vi "SOQPSK Modem.vi"() -> ()   [LabVIEW 2025]
uses:
  chdr/CHDR Header Layout.ctl
  <vilib>/Platform/TimedLoop/XDataNode/timing_clust.ctl
  <vilib>/Platform/TimedLoop/XDataNode/nitl_modes.ctl
  <vilib>/Platform/TimedLoop/XDataNode/wakeup.ctl
  <vilib>/DLsc/v1/FPGA/DLsc/Endpoint/Data Transfer Type.ctl
  <vilib>/DLsc/v1/FPGA/Aurora 64b66b/Aurora Port Identifier.ctl
  Shared/Public/Demodulation Control.ctl
  <vilib>/rvi/Emulation/niFpgaSctlEmulationGetInTimedLoop.vi
  <vilib>/rvi/Emulation/niFpgaEmulationReportErrorSimple.vi
  <vilib>/rvi/Emulation/niFpgaGetClockAttributes.vi
  <vilib>/rvi/Emulation/niFpgaCriticalErrorInLSC.vi
  <vilib>/rvi/Emulation/niFpgaProcessEmulError.vi
  <vilib>/eio/utilities/niEioResolveVilibRelativePath.vi
  <vilib>/rvi/interface/RandomDataEmulation/niFpgaRandomDataHandleErrors.vi
  <vilib>/rvi/Emulation/niFpgaEmulationIsFPGAContextNoSignature.vi
  <vilib>/rvi/errors/niFpgaSetErrorForExecOnDevCompSimple.vi
  <vilib>/rvi/eio/common/nirviEmuReportErrorAndStop.vi
  <vilib>/rvi/DataTransferAndStorage/Container/Common/niFpgaContainerGetUniqueNameForEmu.vi
  <vilib>/rvi/FIFO/Fifo_Resource/nirvififoEmulationSetSize.vi
  <vilib>/rvi/FIFO/Fifo_Resource/nirviFifoEmulationQueueMgr.vi
  <instcachedir>/0/nirviFifoEmulationQueueMgr_E5CAEC123FF24DC58D834DCA3CDAA9B5.lvgen/nirviFifoEmulationQueueMgr_E5CAEC123FF24DC58D834DCA3CDAA9B5_011.vi
  <vilib>/rvi/FIFO/Fifo_Resource/nirvififoEmulationDetermineInputValidOut.vi
  <vilib>/rvi/FIFO/Fifo_Resource/nirvififoEmulationCreateLock.vi
  <vilib>/rvi/FIFO/Fifo_Resource/nirvififoEmulationObtainLock.vi
  <vilib>/rvi/FIFO/Fifo_Resource/nirvififoEmulationReleaseLock.vi
  <vilib>/rvi/occurrence/nirviWaitOnOccurrenceBase.vi
  <vilib>/rvi/errors/nirviReportUnexpectedCaseInternalError.vi
  <vilib>/rvi/errors/nirviReportUnexpectedCaseInternalError (U32).vi
  <vilib>/rvi/interface/RandomDataEmulation/nirviRandomDataMultiElementFPGAFIFO.vi
  <instcachedir>/0/nirviRandomDataMultiElementFPGAFIFO_BE2FF10D3D6E420AB0291A02835C249E.lvgen/nirviRandomDataMultiElementFPGAFIFO_BE2FF10D3D6E420AB0291A02835C249E_001.vi
  <instrlib>/_niInstr/Basic Elements/v1/FPGA/Private/Count Up U32.vi
  <vilib>/rvi/Memory/Memory_Emulation/nirvimemoryFastEmulation.vi
  <vilib>/rvi/Memory/Memory_Emulation/nirvimemoryEmulation.vi
  <vilib>/Utility/error.llb/Clear Errors.vi
  <vilib>/rvi/DataTransferAndStorage/Container/Common/niFpgaContainerSetEmuInfo.vi
  <vilib>/DLsc/v1/FPGA/Aurora 64b66b/Create DX Advanced.vi
  <vilib>/DLsc/v1/FPGA/DLsc/Endpoint/Write Data Stream with Framing 256 Bits.vi
  <vilib>/DLsc/v1/FPGA/DLsc/Endpoint/Read Data Stream with Framing 256 Bits.vi
  <instrlib>/_niInstr/Basic Elements/v1/FPGA/Private/Count Up U64.vi
  <vilib>/Platform/TimedLoop/XDataNode/XDataNode.xnode
  <vilib>/rvi/DataTransferAndStorage/Container/XNode/niFpgaContainer.xnode
  <vilib>/rvi/interface/RandomDataEmulation/nirviRandomDataFpgaReadWriteTemplate.vi
  <vilib>/rvi/FIFO/Fifo_Resource/nirvififoEmulationWrite.vi
  <vilib>/rvi/interface/RandomDataEmulation/nirviRandomDataFpgaMultiElementTemplate.vi
  <vilib>/rvi/FIFO/Fifo_Resource/nirvififoEmulationRead.vi
  <vilib>/rvi/LocalResourceManager/LocalResourceManager.xnode
  <vilib>/DataMovement_sc/v1/FPGA/Buffer U32 8 to 1 SPC/Buffer U32 8 to 1 SPC v1 FPGA.lvclass
  <vilib>/DataMovement_sc/v1/FPGA/Buffer U32 2 to 8 SPC/Buffer U32 2 to 8 SPC v1 FPGA.lvclass
  Shared/BER/FPGA/BER/BER.lvclass
  <vilib>/Platform/TimedLoop/XDataNode/XDNodeRunTimeDep.lvlib
  chdr/CHDR Support.lvlib
  <instrlib>/_niInstr/Basic Elements/v1/FPGA/niInstr Basic Elements v1 FPGA.lvlib
  <vilib>/DataMovement_sc/v1/Shared/Data Types/DMsc Data Types v1 Shared.lvlib
  <instrlib>/_niInstr/FIFO Register Bus/v1/FPGA/niInstr FIFO Register Bus v1 FPGA.lvclass
  <vilib>/DLsc/v1/FPGA/DLsc/Collection/Endpoint Collection.lvclass
  <vilib>/DLsc/v1/FPGA/DLsc/Endpoint/Endpoint.lvclass
  Shared/Modems Shared.lvlib
  Shared/AWGN/FPGA/AWGN FPGA.lvlib
  Shared/SOQPSK Modem Shared.lvlib
  <vilib>/DLsc/v1/FPGA/Aurora 64b66b/DLsc Aurora 64b66b v1 FPGA.lvlib
panel:
  in  "update bit generation.1":bool
  out "last_header.1":T1
  out "last_timestamp.1":u64
  out "error detection.1":T2
  out "header count.1":u64
  in  "reset rx.1":bool
  in  "enable match filter.1":bool
  in  "symmetric filter coefficients .1":T3 {"symmetric filter coefficients[16]" format="%.16g"; "symmetric filter coefficients[0]" format="%.16g"; "symmetric filter coefficients[1]" format="%.16g"; "symmetric filter coefficients[2]" format="%.16g"; "symmetric filter coefficients[3]" format="%.16g"; "symmetric filter coefficients[4]" format="%.16g"; "symmetric filter coefficients[5]" format="%.16g"; "symmetric filter coefficients[6]" format="%.16g"; "symmetric filter coefficients[7]" format="%.16g"; "symmetric filter coefficients[8]" format="%.16g"; "symmetric filter coefficients[9]" format="%.16g"; "symmetric filter coefficients[10]" format="%.16g"; "symmetric filter coefficients[11]" format="%.16g"; "symmetric filter coefficients[12]" format="%.16g"; "symmetric filter coefficients[13]" format="%.16g"; "symmetric filter coefficients[14]" format="%.16g"; "symmetric filter coefficients[15]" format="%.16g"}
  in  "payload length.1":u32
  out "current threshold.1":fxp<+/-,15,15>
  in  "enable aurora debug.1":bool
  in  "preamble.1":i32
  out "demodulated bits overflow.1":bool
  out "aurora debug overflow.1":bool
  out "recovered IQ overflow.1":bool
  in  "demodulation control.1":i16
  out "demodulated bits to BER overflow.1":bool
  out "bit stream length.1":u32
  out "write data stream overflow.1":bool
  in  "reset overflow status.1":bool
  out "modulator error.1":bool
  in  "soqpsk parameters.1":T4
  in  "enable precoder.1":bool
  in  "scaling factor.1":fxp<+,16,0> format="%.16g"
  in  "output type selection.1":u16
  in  "reset modulator.1":bool
  in  "AWGN seeds.1":fxp<+,25,25>[](array[numeric])=[0.0, 0.0]
  in  "enable modulator.1":bool
  in  "header parameters.1":T5
  in  "aurora frame length.1":u16
  in  "reset tx.1":bool
  in  "update bit generation.0":bool
  out "demodulated bits to BER overflow.0":bool
  in  "demodulation control.0":i16
  out "recovered IQ overflow.0":bool
  out "aurora debug overflow.0":bool
  out "demodulated bits overflow.0":bool
  in  "preamble.0":i32
  in  "enable aurora debug.0":bool
  out "current threshold.0":fxp<+/-,15,15>
  in  "payload length.0":u32
  in  "symmetric filter coefficients.0":T3 {"symmetric filter coefficients[16]" format="%.16g"; "symmetric filter coefficients[0]" format="%.16g"; "symmetric filter coefficients[1]" format="%.16g"; "symmetric filter coefficients[2]" format="%.16g"; "symmetric filter coefficients[3]" format="%.16g"; "symmetric filter coefficients[4]" format="%.16g"; "symmetric filter coefficients[5]" format="%.16g"; "symmetric filter coefficients[6]" format="%.16g"; "symmetric filter coefficients[7]" format="%.16g"; "symmetric filter coefficients[8]" format="%.16g"; "symmetric filter coefficients[9]" format="%.16g"; "symmetric filter coefficients[10]" format="%.16g"; "symmetric filter coefficients[11]" format="%.16g"; "symmetric filter coefficients[12]" format="%.16g"; "symmetric filter coefficients[13]" format="%.16g"; "symmetric filter coefficients[14]" format="%.16g"; "symmetric filter coefficients[15]" format="%.16g"}
  in  "enable match filter.0":bool
  in  "enable modulator.0":bool
  in  "AWGN seeds.0":fxp<+,25,25>[](array[numeric])=[0.0, 0.0]
  in  "reset modulator.0":bool
  in  "output type selection.0":u16
  in  "scaling factor.0":fxp<+,16,0> format="%.16g"
  in  "enable precoder.0":bool
  in  "soqpsk parameters.0":T4
  out "modulator error":bool
  in  "reset overflow status.0":bool
  out "write data stream overflow":bool
  out "bit stream length.0":u32
  out "fifo reg bus status 0":u32
  out "fifo reg bus data 0":u64
  in  "fifo reg bus ctrl 0":u32
  in  "reset rx.0":bool
  out "header count.0":u64
  out "error detection.0":T2
  out "last_timestamp.0":u64
  out "last_header.0":T1
  in  "reset tx.0":bool
  in  "aurora frame length.0":u16
  in  "header parameters.0":T5
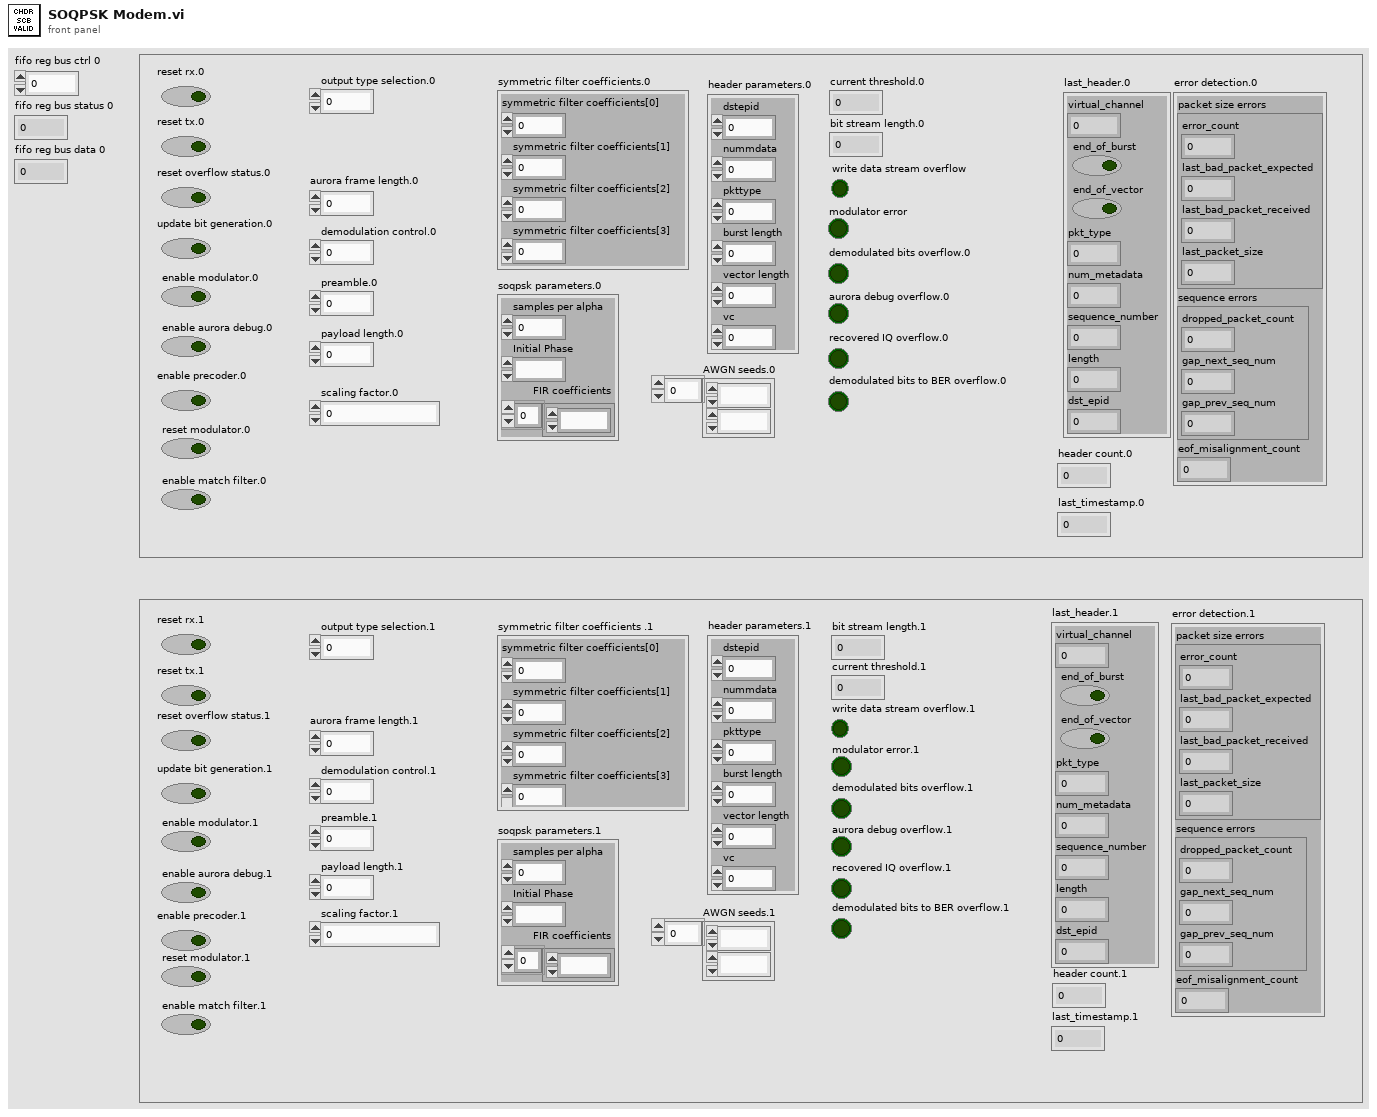
[diagram p1: front panel]
types:
  T1 = typedef "CHDR Support.lvlib/CHDR Header Layout.ctl" = cluster{"virtual_channel":fxp<+,6,6>, "end_of_burst":bool, "end_of_vector":bool, "pkt_type":fxp<+,3,3>, "num_metadata":fxp<+,5,5>, "sequence_number":u16, "length":u16, "dst_epid":u16}
  T2 = cluster{"packet size errors":cluster{"error_count":u64, "last_bad_packet_expected":u16, "last_bad_packet_received":u16, "last_packet_size":u16}, "sequence errors":cluster{"dropped_packet_count":u64, "gap_next_seq_num":u16, "gap_prev_seq_num":u16}, "eof_misalignment_count":u64}
  T3 = cluster{"symmetric filter coefficients[0]":fxp<+/-,16,1>, "symmetric filter coefficients[1]":fxp<+/-,16,1>, "symmetric filter coefficients[2]":fxp<+/-,16,1>, "symmetric filter coefficients[3]":fxp<+/-,16,1>, "symmetric filter coefficients[4]":fxp<+/-,16,1>, "symmetric filter coefficients[5]":fxp<+/-,16,1>, "symmetric filter coefficients[6]":fxp<+/-,16,1>, "symmetric filter coefficients[7]":fxp<+/-,16,1>, "symmetric filter coefficients[8]":fxp<+/-,16,1>, "symmetric filter coefficients[9]":fxp<+/-,16,1>, "symmetric filter coefficients[10]":fxp<+/-,16,1>, "symmetric filter coefficients[11]":fxp<+/-,16,1>, "symmetric filter coefficients[12]":fxp<+/-,16,1>, "symmetric filter coefficients[13]":fxp<+/-,16,1>, "symmetric filter coefficients[14]":fxp<+/-,16,1>, "symmetric filter coefficients[15]":fxp<+/-,16,1>, "symmetric filter coefficients[16]":fxp<+/-,16,1>}
  T4 = cluster{"samples per alpha":u8, "Initial Phase":fxp<+/-,24,1>, "FIR coefficients":fxp<+/-,24,1>[]}
  T5 = cluster{"dstepid":u16, "nummdata":fxp<+,5,5>, "pkttype":fxp<+,3,3>, "burst length":u16, "vector length":u16, "vc":fxp<+,6,6>}
  T6 = typedef "DLsc v1 FPGA.lvlib/Endpoint.lvclass/Data Transfer Type.ctl" = enum16{"u32 1spc", "u32 2spc", "u32 4spc", "u32 8spc", "u32 16spc", "u32 32spc"}
  T7 = typedef "DLsc Aurora 64b66b v1 FPGA.lvlib/Aurora Port Identifier.ctl" = enum16{"Port 0", "Port 1", "Port 2", "Port 3", "Port 4", "Port 5", "Port 6", "Port 7", "Port 8", "Port 9", "Port 10", "Port 11", "Ports 0-1", "Ports 2-3", "Ports 4-5", "Ports 6-7", "Ports 8-9", "Ports 10-11", "Ports 0-3", "Ports 4-7", "Ports 8-11"}
  T8 = typedef "XDNodeRunTimeDep.lvlib/timing_clust.ctl" = cluster{"Expected End [f-1]":u64, "Actual End [f-1]":u64, "Finished Late? [f-1]":bool, "Expected End [i-1]":u64, "Actual End [i-1]":u64, "Finished Late? [i-1]":bool, "Expected Start [i]":u64, "Actual Start [i]":u64, "Expected Start [f]":u64, "Actual Start [f]":u64, "Source Name":string, "Structure Name":string, "Period":i64, "Deadline":i64, "Offset":i64, "Start":i64, "Priority":i32, "Timeout":i32, "Mode":T9, "Wakeup Reason":T10, "Error":errorcluster, "Source Type":string, "Secondary Source Type":string, "Global End Time":u64, "Global Start Time":u64, "Frame Duration":u64, "Iteration Duration":u64, "Assigned CPU":i32, "I/O Scan Engine Mode":u32}
  T9 = typedef "XDNodeRunTimeDep.lvlib/nitl_modes.ctl" = enum32{"No Change", "Process missed periods, maintain original phase", "Discard missed periods, maintain original phase", "Process missed periods, ignore original phase", "Discard missed periods, ignore original phase"}
  T10 = typedef "XDNodeRunTimeDep.lvlib/wakeup.ctl" = enum32{"Normal", "Aborted", "Asynchronous wakeup", "Timing source error", "Timed loop error", "Timeout"}
  T11 = typedef "niInstr DSP v1 Shared.lvlib/IQ Data.ctl" = cluster{"I":fxp<+/-,18,1>, "Q":fxp<+/-,18,1>, "overflow":bool}
  T12 = cluster{"dropped_packet_count":u64, "gap_next_seq_num":u16, "gap_prev_seq_num":u16}
  T13 = cluster{"error_count":u64, "last_bad_packet_expected":u16, "last_bad_packet_received":u16, "last_packet_size":u16}
  T14 = typedef "SOQPSK Modem Shared.lvlib/Demodulation Control.ctl" = i16
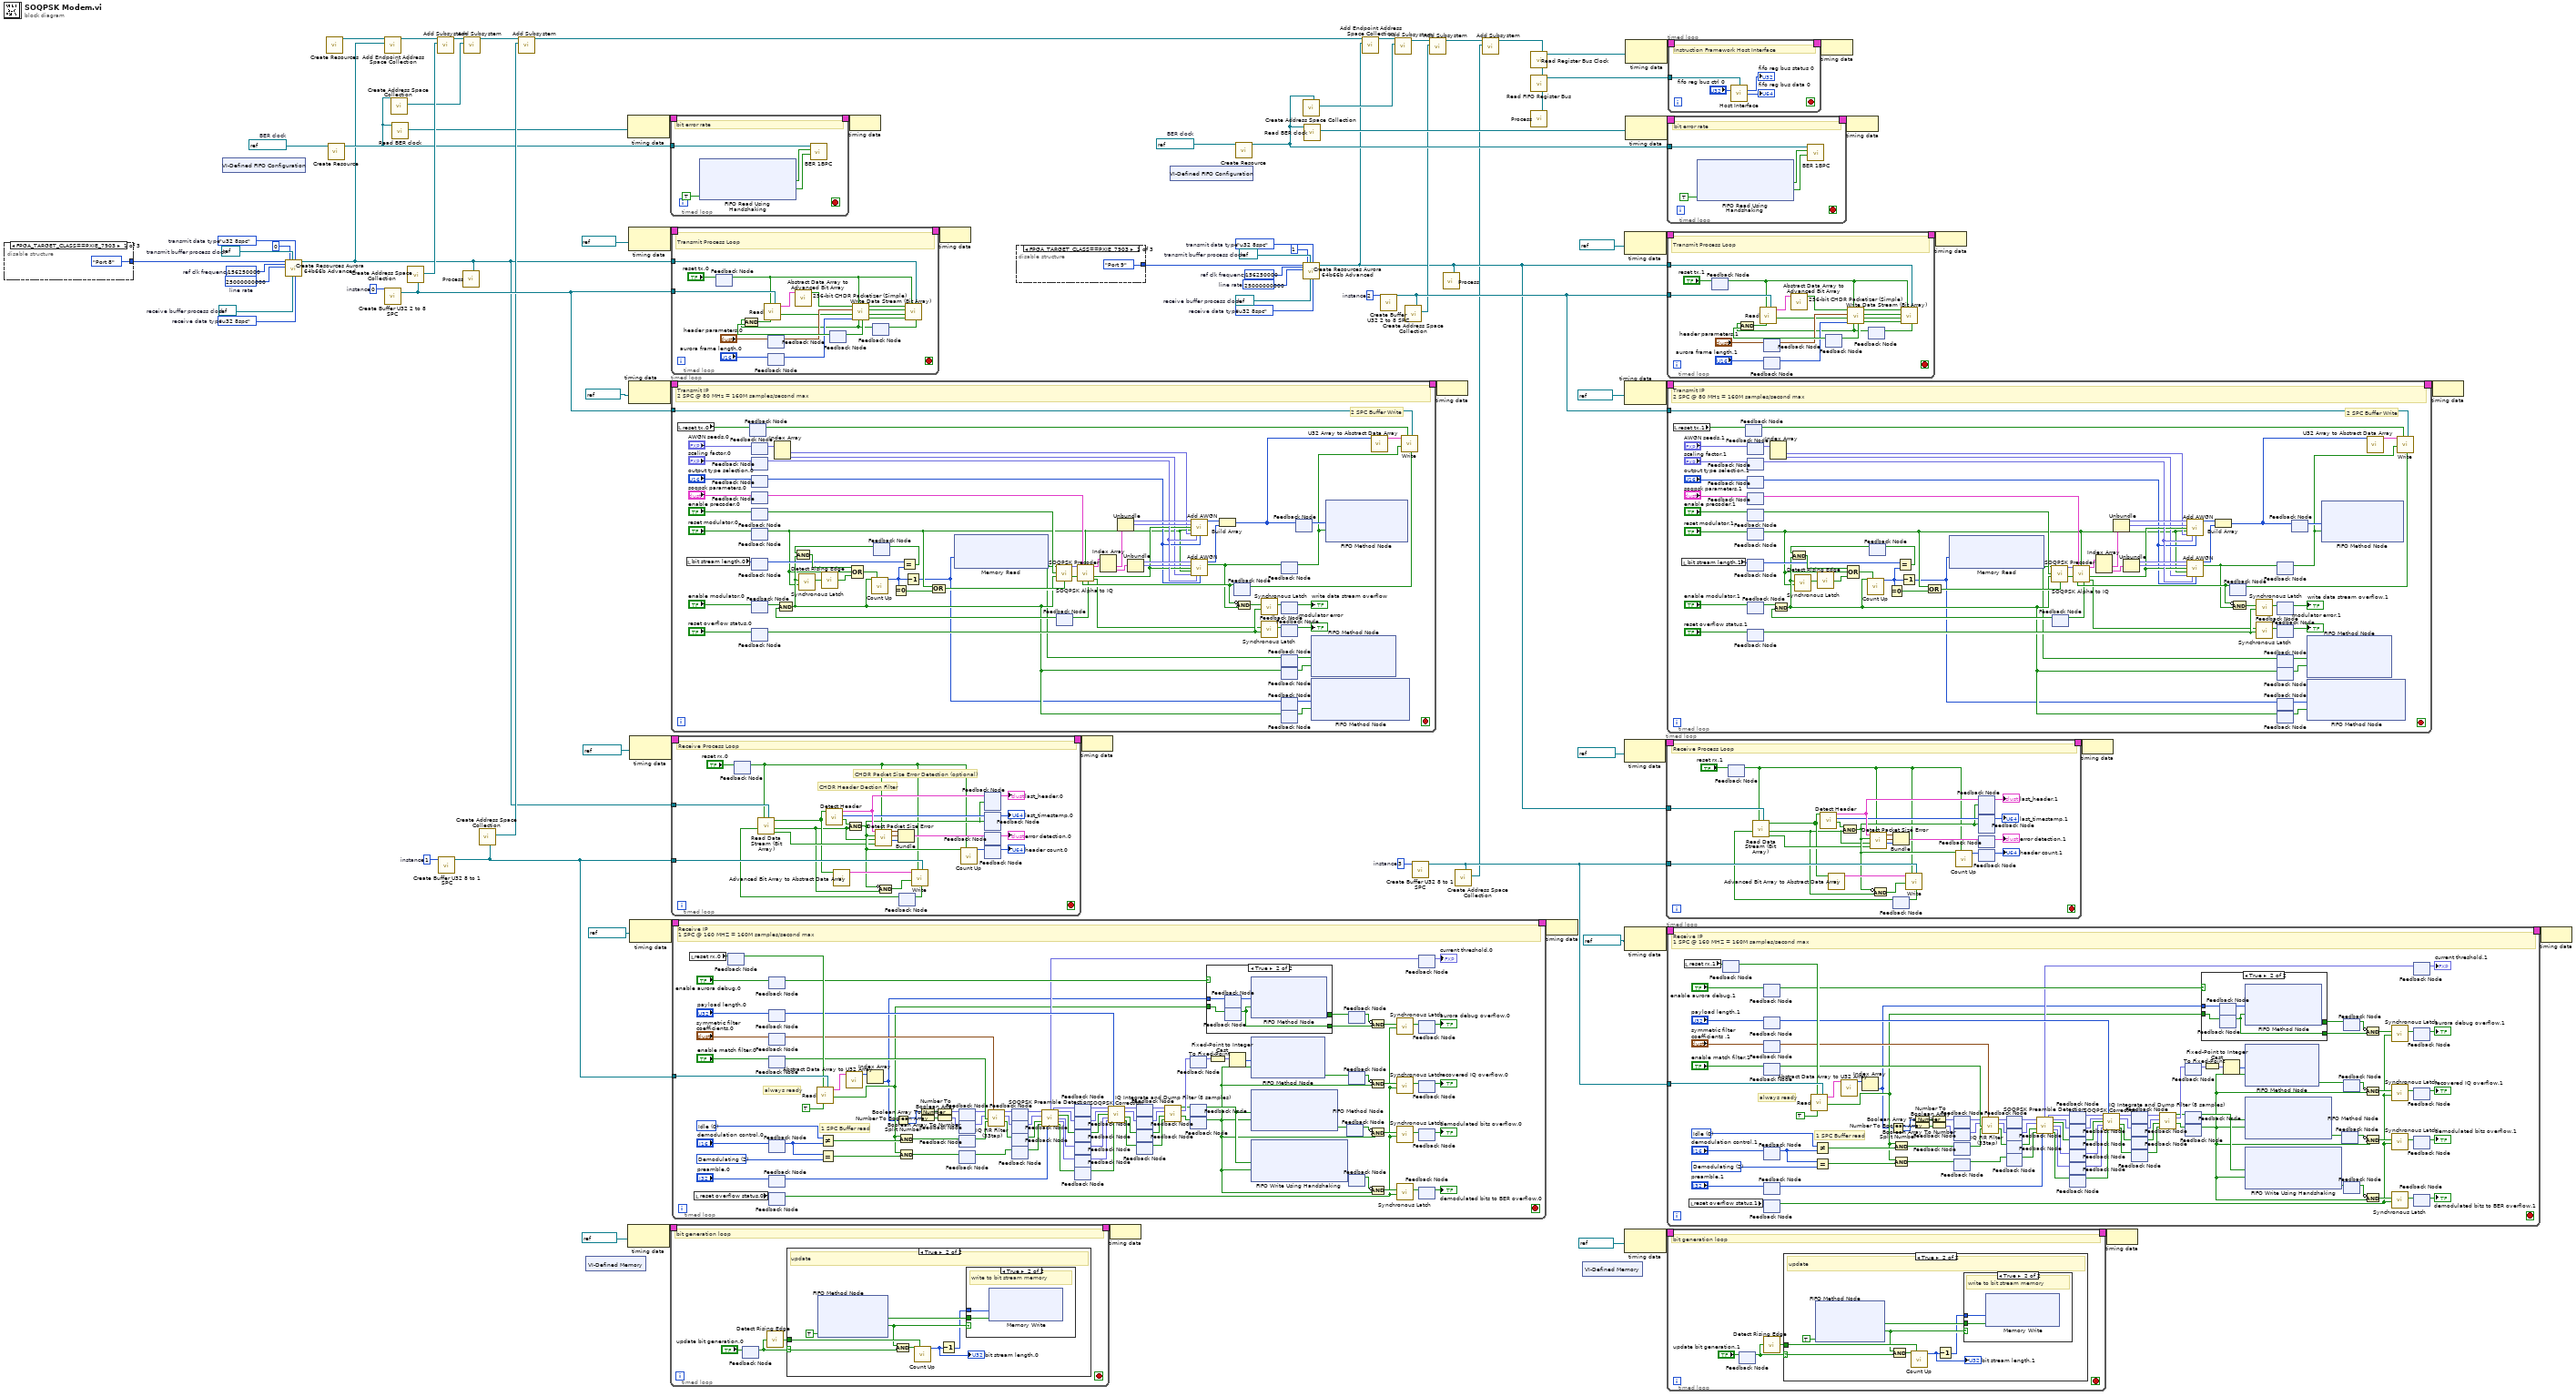
[diagram p0: block diagram]
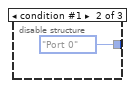
[diagram p2: hidden frame]
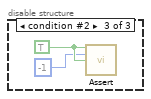
[diagram p3: hidden frame]
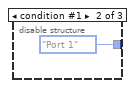
[diagram p4: hidden frame]
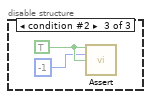
[diagram p5: hidden frame]
diagram:
  w6 = refnum<k21> refnum  # receive buffer process clock
  w9 = Data_Transfer_Type."u32 8spc"  # receive data type
  w4 = refnum<k21> refnum  # transmit buffer process clock
  w5 = Data_Transfer_Type."u32 8spc"  # transmit data type
  w8 = u64 25000000000  # line rate
  w7 = u64 156250000  # ref clk frequency
  w13 = refnum<k21> refnum  # receive buffer process clock
  w16 = Data_Transfer_Type."u32 8spc"  # receive data type
  w11 = refnum<k21> refnum  # transmit buffer process clock
  w12 = Data_Transfer_Type."u32 8spc"  # transmit data type
  w15 = u64 25000000000  # line rate
  w14 = u64 156250000  # ref clk frequency
  w22 = u8 3  # instance
  w39 = u8 2  # instance
  w49 = refnum<k21> "120MHz"  # BER clock
  w60 = refnum<k21> "120MHz"  # BER clock
  w71 = u8 0  # instance
  w72 = u8 1  # instance
  n1 = disable-structure shown="FPGA_TARGET_CLASS==PXIE_7903" {
    disable-tunnel: [Aurora_Port_Identifier."Port 8" ("aurora port identifier") Aurora_Port_Identifier."Port 0" ("aurora port identifier") _] -> w1
    frame condition #0 (active) {
    }
    frame condition #1 {
    }
    frame condition #2 {
      w89 = TRUE ("assert")
      n2 = call <instrlib>:"Assert.vi"("assert"=w89, "error code"=-1, "enable show error"=w89) -> ()  [unwired: 13 in]
    }
  }
  n3 = xnode "VI-Defined FIFO Configuration"() -> ()  [unwired: 1 out]
  n4 = call-poly <vilib>:"Create Resources Aurora 64b66b Advanced.vi"("aurora port identifier"=w1, "ref clk frequency"=w14, "line rate"=w15, "instance (0)"=u8 0, "transmit buffer process clock"=w11, "receive buffer process clock"=w13, "transmit data type"=w12, "receive data type"=w16) -> ("endpoint"=w52:refnum<class "Endpoint.lvclass">)  [unwired: 11 in]
  n5 = call <vilib>:"Create Resources.vi"() -> ("endpoint collection"=w66:refnum<class "Endpoint Collection.lvclass">)  [unwired: 11 in]
  n6 = call "Create Resource.vi"("BER clock"=w60) -> ("BER"=w57:refnum<class "BER.lvclass">)  [unwired: 10 in]
  n7 = call <vilib>:"Create Buffer U32 2 to 8 SPC.vi"("instance (0)"=w71) -> ("buffer u32 2 to 8 spc out"=w74:refnum<class "Buffer U32 2 to 8 SPC v1 FPGA.lvclass">)  [unwired: 10 in]
  n8 = call <vilib>:"Add Endpoint Address Space Collection.vi"("endpoint"=w52, "endpoint collection in"=w66) -> ("endpoint collection out"=w65:refnum<class "Endpoint Collection.lvclass">)  [unwired: 9 in]
  n9 = call-dynamic "Create Address Space Collection.vi"("BER"=w57) -> ("address space collection"=w56:refnum<class "Address Space Collection.lvclass">)  [unwired: 9 in, 1 out]
  n10 = call "Read BER clock.vi"("BER"=w57) -> ("BER clock"=w59:refnum<k21>)  [unwired: 10 in]
  n11 = call-dynamic "Create Address Space Collection.vi"("buffer"=w74) -> ("address space collection"=w64:refnum<class "Address Space Collection.lvclass">)  [unwired: 9 in, 1 out]
  n12 = call <vilib>:"Add Subsystem.vi"("subsystems"=w64, "endpoint collection in"=w65) -> ("endpoint collection out"=w58:refnum<class "Endpoint Collection.lvclass">)  [unwired: 9 in]
  n13 = call <vilib>:"Create Buffer U32 8 to 1 SPC.vi"("instance (0)"=w72) -> ("buffer u32 8 to 1 spc"=w73:refnum<class "Buffer U32 8 to 1 SPC v1 FPGA.lvclass">)  [unwired: 10 in]
  n14 = call <vilib>:"Process.vi"("endpoint"=w52) -> ()  [unwired: 11 in]
  n15 = call <vilib>:"Add Subsystem.vi"("subsystems"=w56, "endpoint collection in"=w58) -> ("endpoint collection out"=w33:refnum<class "Endpoint Collection.lvclass">)  [unwired: 9 in]
  n16 = call-dynamic "Create Address Space Collection.vi"("buffer"=w73) -> ("address space collection"=w63:refnum<class "Address Space Collection.lvclass">)  [unwired: 9 in, 1 out]
  n17 = call <vilib>:"Add Subsystem.vi"("subsystems"=w63, "endpoint collection in"=w33) -> ("endpoint collection out"=w34:refnum<class "Endpoint Collection.lvclass">)  [unwired: 9 in]
  n18 = xnode "VI-Defined Memory"() -> ()  [unwired: 1 out]
  n19 = node-c288(w59) -> (w62:T8)
  n20 = node-c288(refnum<k21> "80MHz" ("Source Name")) -> (w55:T8)
  n21 = node-c288(refnum<k21> "80MHz" ("Source Name")) -> (w85:T8)
  n22 = node-c288(refnum<k21> "80MHz" ("Source Name")) -> (w76:T8)
  n23 = node-c288(refnum<k21> "160MHz" ("Source Name")) -> (w82:T8)
  n24 = node-c288(refnum<k21> "160MHz" ("Source Name")) -> (w79:T8)
  n25 = timed-loop {
    timing: w62 -> [_]
    timing-out: [_] -> w61
    tunnel: w57 -> [w93]
    stop <- _ stop-if-true
    # "bit error rate"
    n26 = xnode ("FIFO Read Using Handshaking")("Ready for Output"=TRUE) -> ("Element"=w92:bool, "Output Valid"=w91:bool)  [unwired: 1 in, 1 out]
    n27 = call "BER 1BPC.vi"("input valid"=w91, "input bits"=w92, "BER"=w93) -> ()  [unwired: 9 in]
  }
  n28 = timed-loop {
    timing: w55 -> [_]
    timing-out: [_] -> w54
    stop <- _ stop-if-true
    # "bit generation loop"
    n29 = feedback #1() -> (w97:bool)  [unwired: 1 in]
    n30 = feedback-in #1("update bit generation.0") -> ()
    n31 = call <instrlib>:"Detect Rising Edge.vi"("signal"=w97) -> ("edge detected"=w96:bool)  [unwired: 14 in]
    n32 = case shown="True" w97 {
      selector: w97 -> [_ w103]
      tunnel: w96 -> [_ w106]
      frame False {
        # "Don't update"
      }
      frame True {
        # "update"
        n33 = xnode ("FIFO Method Node")("Ready for Output"=TRUE) -> ("Element"=w105:bool, "Output Valid"=w101:bool)  [unwired: 1 in, 1 out]
        n34 = Compound Arithmetic op=AND(w101, w103) -> (w102:bool)
        n35 = call-poly <instrlib>:"Count Up.vi"("increment"=w102, "reset"=w106) -> ("count out"=w99:u32)  [unwired: 13 in]
        "bit stream length.0" <- w99
        n36 = Decrement(x=w99) -> (x-1=w100:u32)
        n37 = case shown="True" w101 {
          tunnel: w100 -> [_ w108]
          tunnel: w105 -> [_ w107]
          frame False {
            # "nothing to write"
          }
          frame True {
            # "write to bit stream memory"
            n38 = xnode ("Memory Write")("Address"=w108, "Data"=w107) -> ()  [unwired: 1 in, 1 out]
          }
        }
      }
    }
  }
  n39 = timed-loop {
    timing: w85 -> [_]
    timing-out: [_] -> w84
    tunnel: w74 -> [w119]
    tunnel: w52 -> [w117]
    stop <- _ stop-if-true
    # "Transmit Process Loop"
    n40 = feedback #2() -> (w112:bool)  [unwired: 1 in]
    n41 = feedback-in #2("reset tx.0") -> ()
    n42 = feedback #3() -> (w127:T5)  [unwired: 1 in]
    n43 = feedback-in #3("header parameters.0") -> ()
    n44 = feedback #4() -> (w125:u16)  [unwired: 1 in]
    n45 = feedback-in #4("aurora frame length.0") -> ()
    n46 = feedback #5() -> (w129:bool)  [unwired: 1 in]
    n47 = feedback #6() -> (w111:bool)  [unwired: 1 in]
    n48 = Compound Arithmetic op=AND(w111, w129) -> (w123:bool)
    n49 = call-dynamic "Read.vi"("buffer u32 common"=w119, "ready for output"=w123, "reset"=w112) -> ("output valid"=w120:bool, "data out"=w122:cluster{"data":bool[]}[])  [unwired: 7 in]
    n50 = call <vilib>:"Abstract Data Array to Advanced Bit Array.vi"("data in"=w122) -> ("data"=w121:bool[])  [unwired: 8 in, 2 out]
    n51 = call "256-bit CHDR Packetizer (Simple).vi"("ready for output"=w111, "reset"=w112, "aurora frame length"=w125, "input valid"=w120, "header parameters"=w127, "data"=w121) -> ("tlast"=w114:bool, "output valid"=w115:bool, "tkeep"=w116:bool[], "data out"=w118:bool[], "ready for input"=w130:bool)  [unwired: 1 in]
    n52 = feedback-in #5(w130) -> ()
    n53 = call-poly <vilib>:"Write Data Stream (Bit Array).vi"("endpoint"=w117, "reset"=w112, "end of frame"=w114, "input valid"=w115, "byte enable"=w116, "data"=w118) -> ("ready for input"=w113:bool)  [unwired: 5 in]
    n54 = feedback-in #6(w113) -> ()
  }
  n55 = timed-loop {
    timing: w76 -> [_]
    timing-out: [_] -> w75
    tunnel: w74 -> [w197]
    stop <- _ stop-if-true
    # "2 SPC Buffer Write"
    # "Transmit IP\n2 SPC @ 80 MHz = 160M samples/second max"
    n56 = local read "reset tx.0"() -> (w198:bool)
    n57 = local read "bit stream length.0"() -> (w178:u32)
    n58 = feedback #7() -> (w196:bool)  [unwired: 1 in]
    n59 = feedback-in #7(w198) -> ()
    n60 = feedback #8() -> (w142:fxp<+,25,25>[])  [unwired: 1 in]
    n61 = feedback-in #8("AWGN seeds.0") -> ()
    n62 = feedback #9() -> (w157:fxp<+,16,0>)  [unwired: 1 in]
    n63 = feedback-in #9("scaling factor.0") -> ()
    n64 = feedback #10() -> (w154:u16)  [unwired: 1 in]
    n65 = feedback-in #10("output type selection.0") -> ()
    n66 = feedback #11() -> (w182:T4)  [unwired: 1 in]
    n67 = feedback-in #11("soqpsk parameters.0") -> ()
    n68 = feedback #12() -> (w148:bool)  [unwired: 1 in]
    n69 = feedback-in #12("enable precoder.0") -> ()
    n70 = feedback #13() -> (w141:bool)  [unwired: 1 in]
    n71 = feedback-in #13("reset modulator.0") -> ()
    n72 = feedback #14() -> (w170:u32)  [unwired: 1 in]
    n73 = feedback-in #14(w178) -> ()
    n74 = feedback #15() -> (w139:bool)  [unwired: 1 in]
    n75 = feedback-in #15("enable modulator.0") -> ()
    n76 = feedback #16() -> (w192:bool)  [unwired: 1 in]
    n77 = feedback-in #16("reset overflow status.0") -> ()
    n78 = Index Array(array=w142) -> (element #1=w145:fxp<+,25,25>, element #2=w144:fxp<+,25,25>)  [unwired: 2 in]
    n79 = feedback #17() -> (w172:bool)  [unwired: 1 in]
    n80 = feedback #18() -> (w173:bool)  [unwired: 1 in]
    n81 = Compound Arithmetic op=AND(w139, w173) -> (w150:bool)
    n82 = Compound Arithmetic op=AND(w172, w150) -> (w171:bool)
    n83 = call <instrlib>:"Synchronous Latch.vi"("clear"=w141, "set"=w150) -> ("out"=w169:bool)  [unwired: 9 in]
    n84 = call <instrlib>:"Detect Rising Edge.vi"("signal"=w169) -> ("edge detected"=w168:bool)  [unwired: 14 in]
    n85 = Compound Arithmetic op=OR(w171, w141, w168) -> (w177:bool)
    n86 = call-poly <instrlib>:"Count Up.vi"("increment"=w150, "reset"=w177) -> ("count out"=w167:u32)  [unwired: 13 in]
    n87 = Equal To 0?(x=w167) -> (x = 0?=w194:bool)
    n88 = Equal?(x=w170, y=w167) -> (x = y?=w193:bool)
    n89 = feedback-in #17(w193) -> ()
    n90 = Decrement(x=w167) -> (x-1=w138:u32)
    n91 = Compound Arithmetic op=OR(w141, w194) -> (w166:bool)
    n92 = xnode ("Memory Read")("Address"=w138) -> ("Data"=w137:bool)  [unwired: 1 in, 1 out]
    n93 = call "SOQPSK Precoder.vi"("Bit In"=w137, "enable"=w148, "input valid"=w150, "reset"=w166) -> ("Alpha Out"=w181:fxp<+/-,3,2>, "output valid"=w180:bool)  [unwired: 9 in, 1 out]
    n94 = feedback #19() -> (w186:bool)  [unwired: 1 in]
    n95 = call "SOQPSK Alpha to IQ.vi"("Alpha in"=w181, "SOQPSK Parameters"=w182, "input valid"=w180, "ready for output"=w186, "reset"=w141) -> ("IQ data out"=w187:T11[], "output valid"=w156:bool, "ready for input"=w185:bool, "error"=w175:bool)  [unwired: 5 in, 2 out]
    n96 = feedback-in #18(w185) -> ()
    n97 = Index Array(array=w187) -> (element #1=w165:T11, element #2=w147:T11)  [unwired: 2 in]
    n98 = Unbundle(w165) -> ("I"=w164:fxp<+/-,18,1>, "Q"=w163:fxp<+/-,18,1>)  [unwired: 1 out]
    n99 = Unbundle(w147) -> ("I"=w162:fxp<+/-,18,1>, "Q"=w161:fxp<+/-,18,1>)  [unwired: 1 out]
    n100 = call "Add AWGN.vi"("real"=w164, "img"=w163, "input valid"=w156, "reset"=w141, "seed"=w145, "scaling factor"=w157, "Output Type Selection"=w154) -> ("output with noise"=w160:u32)  [unwired: 7 in, 1 out]
    n101 = call "Add AWGN.vi"("real"=w162, "img"=w161, "input valid"=w156, "reset"=w141, "seed"=w144, "scaling factor"=w157, "Output Type Selection"=w154) -> ("output with noise"=w159:u32, "output valid"=w136:bool)  [unwired: 7 in]
    n102 = Build Array(w160, w159) -> (w134:u32[])
    n103 = Compound Arithmetic op=AND(invert w186, w136) -> (w191:bool)
    n104 = call <instrlib>:"Synchronous Latch.vi"("clear"=w192, "set"=w191) -> ("out"=w189:bool)  [unwired: 9 in]
    n105 = call <instrlib>:"Synchronous Latch.vi"("clear"=w192, "set"=w175) -> ("out"=w174:bool)  [unwired: 9 in]
    n106 = feedback #20() -> (w133:bool)  [unwired: 1 in]
    n107 = feedback-in #20(w136) -> ()
    n108 = feedback #21() -> (→"write data stream overflow":bool)  [unwired: 1 in]
    n109 = feedback-in #21(w189) -> ()
    n110 = feedback #22() -> (→"modulator error":bool)  [unwired: 1 in]
    n111 = feedback-in #22(w174) -> ()
    n112 = feedback #23() -> (w153:bool)  [unwired: 1 in]
    n113 = feedback-in #23(w137) -> ()
    n114 = feedback #24() -> (w152:bool)  [unwired: 1 in]
    n115 = feedback-in #24(w150) -> ()
    n116 = feedback #25() -> (w151:u32)  [unwired: 1 in]
    n117 = feedback-in #25(w138) -> ()
    n118 = feedback #26() -> (w149:bool)  [unwired: 1 in]
    n119 = feedback-in #26(w150) -> ()
    n120 = feedback #27() -> (w176:u32[])  [unwired: 1 in]
    n121 = feedback-in #27(w134) -> ()
    n122 = xnode ("FIFO Method Node")("Element"=w153, "Input Valid"=w152) -> ()  [unwired: 1 in, 2 out]
    n123 = xnode ("FIFO Method Node")("Element"=w151, "Input Valid"=w149) -> ()  [unwired: 1 in, 2 out]
    n124 = xnode ("FIFO Method Node")("Element"=w176, "Input Valid"=w133) -> ()  [unwired: 1 in, 2 out]
    n125 = call <vilib>:"U32 Array to Abstract Data Array.vi"("data in"=w134) -> ("data out"=w195:cluster{"Boolean array":bool[]}[])  [unwired: 10 in]
    n126 = call-dynamic "Write.vi"("buffer u32 common"=w197, "reset"=w196, "input valid"=w133, "data in"=w195) -> ("ready for input"=w135:bool)  [unwired: 7 in]
    n127 = feedback-in #19(w135) -> ()
  }
  n128 = timed-loop {
    timing: w82 -> [_]
    timing-out: [_] -> w81
    tunnel: w73 -> [w215]
    tunnel: w52 -> [w206]
    stop <- _ stop-if-true
    # "CHDR Packet Size Error Detection (optional)"
    # "CHDR Header Dection Filter"
    # "Receive Process Loop"
    n129 = feedback #28() -> (w204:bool)  [unwired: 1 in]
    n130 = feedback-in #28("reset rx.0") -> ()
    n131 = feedback #29() -> (w201:bool)  [unwired: 1 in]
    n132 = call-poly <vilib>:"Read Data Stream (Bit Array).vi"("endpoint"=w206, "reset"=w204, "ready for output"=w201) -> ("end of frame"=w205:bool, "output valid"=w202:bool, "data"=w203:bool[])  [unwired: 5 in, 1 out]
    n133 = call "Detect Header.vi"("input data"=w203) -> ("header detected"=w211:bool, "timestamp"=w209:u64, "chdr_header"=w210:T1)  [unwired: 8 in]
    n134 = call <vilib>:"Advanced Bit Array to Abstract Data Array.vi"("data in"=w203) -> ("data out"=w212:cluster{"Boolean array":bool[]}[])  [unwired: 10 in]
    n135 = Compound Arithmetic op=AND(w211, w202) -> (w208:bool)
    n136 = call "Detect Packet Size Error.vi"("reset_pse"=w204, "end of frame"=w205, "input valid"=w202, "packet_header"=w208, "chdr_header"=w210) -> ("eof_misalignment_count"=w220:u64, "sequence errors"=w221:T12, "packet size errors"=w222:T13)  [unwired: 4 in]
    n137 = Compound Arithmetic op=AND(invert w208, w202) -> (w214:bool)
    n138 = Bundle("packet size errors"=w222, "sequence errors"=w221, "eof_misalignment_count"=w220) -> (w218:T2)  [unwired: 1 in]
    n139 = call-dynamic "Write.vi"("buffer u32 common"=w215, "reset"=w204, "input valid"=w214, "data in"=w212) -> ("ready for input"=w213:bool)  [unwired: 7 in]
    n140 = feedback-in #29(w213) -> ()
    n141 = call-poly <instrlib>:"Count Up.vi"("increment"=w208, "reset"=w204) -> ("count out"=w219:u64)  [unwired: 13 in]
    n142 = feedback #30() -> (→"last_header.0":T1)  [unwired: 1 in]
    n143 = feedback-in #30(w210, w208) -> ()
    n144 = feedback #31() -> (→"last_timestamp.0":u64)  [unwired: 1 in]
    n145 = feedback-in #31(w209, w208) -> ()
    n146 = feedback #32() -> (→"error detection.0":T2)  [unwired: 1 in]
    n147 = feedback-in #32(w218) -> ()
    n148 = feedback #33() -> (→"header count.0":u64)  [unwired: 1 in]
    n149 = feedback-in #33(w219) -> ()
  }
  n150 = timed-loop {
    timing: w79 -> [_]
    timing-out: [_] -> w78
    tunnel: w73 -> [w322]
    stop <- _ stop-if-true
    w305 = T14 2 items=["Idle", "Initial Threshold Detection", "Demodulating"] ("Demodulation Control")
    w307 = T14 0 items=["Idle", "Initial Threshold Detection", "Demodulating"] ("Demodulation Control")
    # "always ready"
    # "1 SPC Buffer read"
    # "Receive IP\n1 SPC @ 160 MHZ = 160M samples/second max"
    n151 = local read "reset rx.0"() -> (w319:bool)
    n152 = local read "reset overflow status.0"() -> (w277:bool)
    n153 = feedback #34() -> (w318:bool)  [unwired: 1 in]
    n154 = feedback-in #34(w319) -> ()
    n155 = feedback #35() -> (w301:bool)  [unwired: 1 in]
    n156 = feedback-in #35("enable aurora debug.0") -> ()
    n157 = feedback #36() -> (w284:u32)  [unwired: 1 in]
    n158 = feedback-in #36("payload length.0") -> ()
    n159 = feedback #37() -> (w310:T3)  [unwired: 1 in]
    n160 = feedback-in #37("symmetric filter coefficients.0") -> ()
    n161 = feedback #38() -> (w312:bool)  [unwired: 1 in]
    n162 = feedback-in #38("enable match filter.0") -> ()
    n163 = feedback #39() -> (w304:i16)  [unwired: 1 in]
    n164 = feedback-in #39("demodulation control.0") -> ()
    n165 = feedback #40() -> (w285:i32)  [unwired: 1 in]
    n166 = feedback-in #40("preamble.0") -> ()
    n167 = feedback #41() -> (w230:bool)  [unwired: 1 in]
    n168 = feedback-in #41(w277) -> ()
    n169 = call-dynamic "Read.vi"("buffer u32 common"=w322, "ready for output"=TRUE, "reset"=w318) -> ("output valid"=w229:bool, "data out"=w320:cluster{"data":bool[]}[])  [unwired: 7 in]
    n170 = Not Equal?(x=w307, y=w304) -> (x != y?=w306:bool)
    n171 = Equal?(x=w304, y=w305) -> (x = y?=w303:bool)
    n172 = call <vilib>:"Abstract Data Array to U32 Array.vi"("data in"=w320) -> ("data out"=w227:u32[])  [unwired: 10 in]
    n173 = Index Array(array=w227) -> (element=w228:u32)  [unwired: 1 in]
    n174 = Split Number(x=w228) -> (hi(x)=w314:u16, lo(x)=w315:u16)
    n175 = Compound Arithmetic op=AND(w229, w306) -> (w272:bool)
    n176 = Compound Arithmetic op=AND(w229, w303) -> (w270:bool)
    n177 = Number To Boolean Array(number=w315) -> (Boolean array=w316:bool[])
    n178 = Number To Boolean Array(number=w314) -> (Boolean array=w317:bool[])
    n179 = Boolean Array To Number(Boolean array=w316) -> (number=w276:fxp<+/-,16,1>)
    n180 = Boolean Array To Number(Boolean array=w317) -> (number=w274:fxp<+/-,16,1>)
    n181 = feedback #42() -> (w275:fxp<+/-,16,1>)  [unwired: 1 in]
    n182 = feedback-in #42(w276) -> ()
    n183 = feedback #43() -> (w273:fxp<+/-,16,1>)  [unwired: 1 in]
    n184 = feedback-in #43(w274) -> ()
    n185 = feedback #44() -> (w271:bool)  [unwired: 1 in]
    n186 = feedback-in #44(w272) -> ()
    n187 = feedback #45() -> (w245:bool)  [unwired: 1 in]
    n188 = feedback-in #45(w270) -> ()
    n189 = call "IQ FIR Filter (33tap).vi"("I data in"=w275, "symmetric filter coefficients"=w310, "Q data in"=w273, "enable"=w312, "input valid"=w271) -> ("I filtered output"=w243:fxp<+/-,16,2>, "Q filtered output"=w241:fxp<+/-,16,2>, "output valid"=w244:bool)  [unwired: 8 in]
    n190 = feedback #46() -> (w242:fxp<+/-,16,2>)  [unwired: 1 in]
    n191 = feedback-in #46(w243) -> ()
    n192 = feedback #47() -> (w238:fxp<+/-,16,2>)  [unwired: 1 in]
    n193 = feedback-in #47(w241) -> ()
    n194 = feedback #48() -> (w239:bool)  [unwired: 1 in]
    n195 = feedback-in #48(w244) -> ()
    n196 = feedback #49() -> (w240:bool)  [unwired: 1 in]
    n197 = feedback-in #49(w245) -> ()
    n198 = call "SOQPSK Preamble Detection.vi"("x real in"=w242, "x im in"=w238, "input valid"=w239, "enable"=w240, "Preamble"=w285) -> ("current threshold"=w279:fxp<+/-,15,15>, "r after preamble"=w247:fxp<+/-,16,1>, "img after preamble"=w249:fxp<+/-,16,1>, "phase valid"=w251:bool, "frequency offset estimation"=w253:fxp<+/-,25,-7>, "phase estimation"=w255:fxp<+/-,24,2>, "estimation valid"=w257:bool)  [unwired: 3 in, 1 out]
    n199 = feedback #50() -> (w246:fxp<+/-,16,1>)  [unwired: 1 in]
    n200 = feedback-in #50(w247) -> ()
    n201 = feedback #51() -> (w248:fxp<+/-,16,1>)  [unwired: 1 in]
    n202 = feedback-in #51(w249) -> ()
    n203 = feedback #52() -> (w250:bool)  [unwired: 1 in]
    n204 = feedback-in #52(w251) -> ()
    n205 = feedback #53() -> (w252:fxp<+/-,25,-7>)  [unwired: 1 in]
    n206 = feedback-in #53(w253) -> ()
    n207 = feedback #54() -> (w254:fxp<+/-,24,2>)  [unwired: 1 in]
    n208 = feedback-in #54(w255) -> ()
    n209 = feedback #55() -> (w256:bool)  [unwired: 1 in]
    n210 = feedback-in #55(w257) -> ()
    n211 = call "SOQPSK Correction.vi"("real input"=w246, "frame length"=w284, "img input"=w248, "input valid"=w250, "frequency offset estimation"=w252, "phase estimation"=w254, "estimation valid"=w256) -> ("real output"=w263:fxp<+/-,33,4>, "img output"=w261:fxp<+/-,33,4>, "output valid"=w260:bool, "reset for IDF"=w265:bool)  [unwired: 5 in]
    n212 = feedback #56() -> (w262:fxp<+/-,33,4>)  [unwired: 1 in]
    n213 = feedback-in #56(w263) -> ()
    n214 = feedback #57() -> (w259:fxp<+/-,33,4>)  [unwired: 1 in]
    n215 = feedback-in #57(w261) -> ()
    n216 = feedback #58() -> (w258:bool)  [unwired: 1 in]
    n217 = feedback-in #58(w260) -> ()
    n218 = feedback #59() -> (w264:bool)  [unwired: 1 in]
    n219 = feedback-in #59(w265) -> ()
    n220 = call "IQ Integrate and Dump Filter (8 samples).vi"("reset"=w264, "input valid"=w258, "img"=w259, "real"=w262) -> ("output valid"=w266:bool, "output"=w269:fxp<+/-,36,7>, "output bit"=w267:bool)  [unwired: 5 in]
    n221 = feedback #60() -> (w268:fxp<+/-,36,7>)  [unwired: 1 in]
    n222 = feedback-in #60(w269) -> ()
    n223 = feedback #61() -> (w237:bool)  [unwired: 1 in]
    n224 = feedback-in #61(w267) -> ()
    n225 = feedback #62() -> (w231:bool)  [unwired: 1 in]
    n226 = feedback-in #62(w266) -> ()
    n227 = case shown="True" w301 {
      tunnel: w228 -> [_ w324]
      tunnel: w229 -> [_ w326]
      tunnel: [_ w327] -> w292
      tunnel: [_ w325] -> w291
      frame False {
      }
      frame True {
        n228 = feedback #63() -> (w323:u32)  [unwired: 1 in]
        n229 = feedback-in #63(w324) -> ()
        n230 = feedback #64() -> (w325:bool)  [unwired: 1 in]
        n231 = feedback-in #64(w326) -> ()
        n232 = xnode ("FIFO Method Node")("Element"=w323, "Input Valid"=w325) -> ("Ready for Input"=w327:bool)  [unwired: 1 in, 1 out]
      }
    }
    n233 = To Fixed-Point(number=w268) -> (fixed-point=w283:fxp<+/-,32,7>)  [unwired: 1 in]
    n234 = Fixed-Point to Integer Cast(1:w283) -> (0:w282:i32)
    n235 = xnode ("FIFO Method Node")("Element"=w282, "Input Valid"=w231) -> ("Ready for Input"=w281:bool)  [unwired: 1 in, 1 out]
    n236 = xnode ("FIFO Method Node")("Element"=w237, "Input Valid"=w231) -> ("Ready for Input"=w280:bool)  [unwired: 1 in, 1 out]
    n237 = xnode ("FIFO Write Using Handshaking")("Element"=w237, "Input Valid"=w231) -> ("Ready for Input"=w232:bool)  [unwired: 1 in, 1 out]
    n238 = feedback #65() -> (w299:bool)  [unwired: 1 in]
    n239 = feedback-in #65(w280) -> ()
    n240 = feedback #66() -> (w295:bool)  [unwired: 1 in]
    n241 = feedback-in #66(w292) -> ()
    n242 = feedback #67() -> (w286:bool)  [unwired: 1 in]
    n243 = feedback-in #67(w281) -> ()
    n244 = feedback #68() -> (w233:bool)  [unwired: 1 in]
    n245 = feedback-in #68(w232) -> ()
    n246 = Compound Arithmetic op=AND(invert w295, w291) -> (w294:bool)
    n247 = Compound Arithmetic op=AND(invert w286, w231) -> (w287:bool)
    n248 = Compound Arithmetic op=AND(invert w299, w231) -> (w298:bool)
    n249 = Compound Arithmetic op=AND(invert w233, w231) -> (w234:bool)
    n250 = call <instrlib>:"Synchronous Latch.vi"("clear"=w230, "set"=w294) -> ("out"=w293:bool)  [unwired: 9 in]
    n251 = call <instrlib>:"Synchronous Latch.vi"("clear"=w230, "set"=w287) -> ("out"=w288:bool)  [unwired: 9 in]
    n252 = call <instrlib>:"Synchronous Latch.vi"("clear"=w230, "set"=w298) -> ("out"=w297:bool)  [unwired: 9 in]
    n253 = call <instrlib>:"Synchronous Latch.vi"("clear"=w230, "set"=w234) -> ("out"=w235:bool)  [unwired: 9 in]
    n254 = feedback #69() -> (→"current threshold.0":fxp<+/-,15,15>)  [unwired: 1 in]
    n255 = feedback-in #69(w279) -> ()
    n256 = feedback #70() -> (→"aurora debug overflow.0":bool)  [unwired: 1 in]
    n257 = feedback-in #70(w293) -> ()
    n258 = feedback #71() -> (→"recovered IQ overflow.0":bool)  [unwired: 1 in]
    n259 = feedback-in #71(w288) -> ()
    n260 = feedback #72() -> (→"demodulated bits overflow.0":bool)  [unwired: 1 in]
    n261 = feedback-in #72(w297) -> ()
    n262 = feedback #73() -> (→"demodulated bits to BER overflow.0":bool)  [unwired: 1 in]
    n263 = feedback-in #73(w235) -> ()
  }
  n264 = node-c288(w61) -> ()
  n265 = node-c288(w84) -> ()
  n266 = disable-structure shown="FPGA_TARGET_CLASS==PXIE_7903" {
    disable-tunnel: [Aurora_Port_Identifier."Port 9" ("aurora port identifier") Aurora_Port_Identifier."Port 1" ("aurora port identifier") _] -> w2
    frame condition #0 (active) {
    }
    frame condition #1 {
    }
    frame condition #2 {
      w333 = TRUE ("assert")
      n267 = call <instrlib>:"Assert.vi"("assert"=w333, "error code"=-1, "enable show error"=w333) -> ()  [unwired: 13 in]
    }
  }
  n268 = node-c288(w81) -> ()
  n269 = node-c288(w54) -> ()
  n270 = xnode "VI-Defined FIFO Configuration"() -> ()  [unwired: 1 out]
  n271 = call "Create Resource.vi"("BER clock"=w49) -> ("BER"=w48:refnum<class "BER.lvclass">)  [unwired: 10 in]
  n272 = call-dynamic "Create Address Space Collection.vi"("BER"=w48) -> ("address space collection"=w30:refnum<class "Address Space Collection.lvclass">)  [unwired: 9 in, 1 out]
  n273 = call-poly <vilib>:"Create Resources Aurora 64b66b Advanced.vi"("aurora port identifier"=w2, "ref clk frequency"=w7, "line rate"=w8, "instance (0)"=u8 1, "transmit buffer process clock"=w4, "receive buffer process clock"=w6, "transmit data type"=w5, "receive data type"=w9) -> ("endpoint"=w21:refnum<class "Endpoint.lvclass">)  [unwired: 11 in]
  n274 = call "Read BER clock.vi"("BER"=w48) -> ("BER clock"=w47:refnum<k21>)  [unwired: 10 in]
  n275 = call <vilib>:"Add Endpoint Address Space Collection.vi"("endpoint"=w21, "endpoint collection in"=w34) -> ("endpoint collection out"=w32:refnum<class "Endpoint Collection.lvclass">)  [unwired: 9 in]
  n276 = call <vilib>:"Create Buffer U32 2 to 8 SPC.vi"("instance (0)"=w39) -> ("buffer u32 2 to 8 spc out"=w40:refnum<class "Buffer U32 2 to 8 SPC v1 FPGA.lvclass">)  [unwired: 10 in]
  n277 = call <vilib>:"Add Subsystem.vi"("subsystems"=w30, "endpoint collection in"=w32) -> ("endpoint collection out"=w31:refnum<class "Endpoint Collection.lvclass">)  [unwired: 9 in]
  n278 = call-dynamic "Create Address Space Collection.vi"("buffer"=w40) -> ("address space collection"=w37:refnum<class "Address Space Collection.lvclass">)  [unwired: 9 in, 1 out]
  n279 = call <vilib>:"Create Buffer U32 8 to 1 SPC.vi"("instance (0)"=w22) -> ("buffer u32 8 to 1 spc"=w23:refnum<class "Buffer U32 8 to 1 SPC v1 FPGA.lvclass">)  [unwired: 10 in]
  n280 = call <vilib>:"Add Subsystem.vi"("subsystems"=w37, "endpoint collection in"=w31) -> ("endpoint collection out"=w36:refnum<class "Endpoint Collection.lvclass">)  [unwired: 9 in]
  n281 = node-c288(w75) -> ()
  n282 = call <vilib>:"Process.vi"("endpoint"=w21) -> ()  [unwired: 11 in]
  n283 = call-dynamic "Create Address Space Collection.vi"("buffer"=w23) -> ("address space collection"=w20:refnum<class "Address Space Collection.lvclass">)  [unwired: 9 in, 1 out]
  n284 = call <vilib>:"Add Subsystem.vi"("subsystems"=w20, "endpoint collection in"=w36) -> ("endpoint collection out"=w35:refnum<class "Endpoint Collection.lvclass">)  [unwired: 9 in]
  n285 = call <vilib>:"Read Register Bus Clock.vi"("endpoint collection"=w35) -> ("register bus clock"=w67:refnum<k21>)  [unwired: 10 in]
  n286 = call <vilib>:"Read FIFO Register Bus.vi"("endpoint collection"=w35) -> ("fifo register bus"=w68:refnum<class "niInstr FIFO Register Bus v1 FPGA.lvclass">)  [unwired: 10 in]
  n287 = call <vilib>:"Process.vi"("endpoint collection"=w35) -> ()  [unwired: 11 in]
  n288 = node-c288(w78) -> ()
  n289 = xnode "VI-Defined Memory"() -> ()  [unwired: 1 out]
  n290 = node-c288(refnum<k21> "160MHz" ("Source Name")) -> (w27:T8)
  n291 = node-c288(refnum<k21> "80MHz" ("Source Name")) -> (w45:T8)
  n292 = node-c288(refnum<k21> "80MHz" ("Source Name")) -> (w43:T8)
  n293 = node-c288(refnum<k21> "160MHz" ("Source Name")) -> (w29:T8)
  n294 = node-c288(refnum<k21> "80MHz" ("Source Name")) -> (w19:T8)
  n295 = node-c288(w47) -> (w51:T8)
  n296 = node-c288(w67) -> (w70:T8)
  n297 = timed-loop {
    timing: w27 -> [_]
    timing-out: [_] -> w26
    tunnel: w23 -> [w348]
    tunnel: w21 -> [w339]
    stop <- _ stop-if-true
    # "Receive Process Loop"
    n298 = feedback #74() -> (w337:bool)  [unwired: 1 in]
    n299 = feedback-in #74("reset rx.1") -> ()
    n300 = feedback #75() -> (w334:bool)  [unwired: 1 in]
    n301 = call-poly <vilib>:"Read Data Stream (Bit Array).vi"("endpoint"=w339, "reset"=w337, "ready for output"=w334) -> ("end of frame"=w338:bool, "output valid"=w335:bool, "data"=w336:bool[])  [unwired: 5 in, 1 out]
    n302 = call "Detect Header.vi"("input data"=w336) -> ("header detected"=w344:bool, "timestamp"=w342:u64, "chdr_header"=w343:T1)  [unwired: 8 in]
    n303 = call <vilib>:"Advanced Bit Array to Abstract Data Array.vi"("data in"=w336) -> ("data out"=w345:cluster{"Boolean array":bool[]}[])  [unwired: 10 in]
    n304 = Compound Arithmetic op=AND(w344, w335) -> (w341:bool)
    n305 = call "Detect Packet Size Error.vi"("reset_pse"=w337, "end of frame"=w338, "input valid"=w335, "packet_header"=w341, "chdr_header"=w343) -> ("eof_misalignment_count"=w353:u64, "sequence errors"=w354:T12, "packet size errors"=w355:T13)  [unwired: 4 in]
    n306 = Compound Arithmetic op=AND(invert w341, w335) -> (w347:bool)
    n307 = Bundle("packet size errors"=w355, "sequence errors"=w354, "eof_misalignment_count"=w353) -> (w351:T2)  [unwired: 1 in]
    n308 = call-dynamic "Write.vi"("buffer u32 common"=w348, "reset"=w337, "input valid"=w347, "data in"=w345) -> ("ready for input"=w346:bool)  [unwired: 7 in]
    n309 = feedback-in #75(w346) -> ()
    n310 = call-poly <instrlib>:"Count Up.vi"("increment"=w341, "reset"=w337) -> ("count out"=w352:u64)  [unwired: 13 in]
    n311 = feedback #76() -> (→"last_header.1":T1)  [unwired: 1 in]
    n312 = feedback-in #76(w343, w341) -> ()
    n313 = feedback #77() -> (→"last_timestamp.1":u64)  [unwired: 1 in]
    n314 = feedback-in #77(w342, w341) -> ()
    n315 = feedback #78() -> (→"error detection.1":T2)  [unwired: 1 in]
    n316 = feedback-in #78(w351) -> ()
    n317 = feedback #79() -> (→"header count.1":u64)  [unwired: 1 in]
    n318 = feedback-in #79(w352) -> ()
  }
  n319 = timed-loop {
    timing: w45 -> [_]
    timing-out: [_] -> w44
    tunnel: w40 -> [w368]
    tunnel: w21 -> [w366]
    stop <- _ stop-if-true
    # "Transmit Process Loop"
    n320 = feedback #80() -> (w361:bool)  [unwired: 1 in]
    n321 = feedback-in #80("reset tx.1") -> ()
    n322 = feedback #81() -> (w376:T5)  [unwired: 1 in]
    n323 = feedback-in #81("header parameters.1") -> ()
    n324 = feedback #82() -> (w374:u16)  [unwired: 1 in]
    n325 = feedback-in #82("aurora frame length.1") -> ()
    n326 = feedback #83() -> (w378:bool)  [unwired: 1 in]
    n327 = feedback #84() -> (w360:bool)  [unwired: 1 in]
    n328 = Compound Arithmetic op=AND(w360, w378) -> (w372:bool)
    n329 = call-dynamic "Read.vi"("buffer u32 common"=w368, "ready for output"=w372, "reset"=w361) -> ("output valid"=w369:bool, "data out"=w371:cluster{"data":bool[]}[])  [unwired: 7 in]
    n330 = call <vilib>:"Abstract Data Array to Advanced Bit Array.vi"("data in"=w371) -> ("data"=w370:bool[])  [unwired: 8 in, 2 out]
    n331 = call "256-bit CHDR Packetizer (Simple).vi"("ready for output"=w360, "reset"=w361, "aurora frame length"=w374, "input valid"=w369, "header parameters"=w376, "data"=w370) -> ("tlast"=w363:bool, "output valid"=w364:bool, "tkeep"=w365:bool[], "data out"=w367:bool[], "ready for input"=w379:bool)  [unwired: 1 in]
    n332 = feedback-in #83(w379) -> ()
    n333 = call-poly <vilib>:"Write Data Stream (Bit Array).vi"("endpoint"=w366, "reset"=w361, "end of frame"=w363, "input valid"=w364, "byte enable"=w365, "data"=w367) -> ("ready for input"=w362:bool)  [unwired: 5 in]
    n334 = feedback-in #84(w362) -> ()
  }
  n335 = timed-loop {
    timing: w43 -> [_]
    timing-out: [_] -> w42
    tunnel: w40 -> [w446]
    stop <- _ stop-if-true
    # "2 SPC Buffer Write"
    # "Transmit IP\n2 SPC @ 80 MHz = 160M samples/second max"
    n336 = local read "reset tx.1"() -> (w447:bool)
    n337 = local read "bit stream length.1"() -> (w427:u32)
    n338 = feedback #85() -> (w445:bool)  [unwired: 1 in]
    n339 = feedback-in #85(w447) -> ()
    n340 = feedback #86() -> (w391:fxp<+,25,25>[])  [unwired: 1 in]
    n341 = feedback-in #86("AWGN seeds.1") -> ()
    n342 = feedback #87() -> (w406:fxp<+,16,0>)  [unwired: 1 in]
    n343 = feedback-in #87("scaling factor.1") -> ()
    n344 = feedback #88() -> (w403:u16)  [unwired: 1 in]
    n345 = feedback-in #88("output type selection.1") -> ()
    n346 = feedback #89() -> (w431:T4)  [unwired: 1 in]
    n347 = feedback-in #89("soqpsk parameters.1") -> ()
    n348 = feedback #90() -> (w397:bool)  [unwired: 1 in]
    n349 = feedback-in #90("enable precoder.1") -> ()
    n350 = feedback #91() -> (w390:bool)  [unwired: 1 in]
    n351 = feedback-in #91("reset modulator.1") -> ()
    n352 = feedback #92() -> (w419:u32)  [unwired: 1 in]
    n353 = feedback-in #92(w427) -> ()
    n354 = feedback #93() -> (w388:bool)  [unwired: 1 in]
    n355 = feedback-in #93("enable modulator.1") -> ()
    n356 = feedback #94() -> (w441:bool)  [unwired: 1 in]
    n357 = feedback-in #94("reset overflow status.1") -> ()
    n358 = Index Array(array=w391) -> (element #1=w394:fxp<+,25,25>, element #2=w393:fxp<+,25,25>)  [unwired: 2 in]
    n359 = feedback #95() -> (w421:bool)  [unwired: 1 in]
    n360 = feedback #96() -> (w422:bool)  [unwired: 1 in]
    n361 = Compound Arithmetic op=AND(w388, w422) -> (w399:bool)
    n362 = Compound Arithmetic op=AND(w421, w399) -> (w420:bool)
    n363 = call <instrlib>:"Synchronous Latch.vi"("clear"=w390, "set"=w399) -> ("out"=w418:bool)  [unwired: 9 in]
    n364 = call <instrlib>:"Detect Rising Edge.vi"("signal"=w418) -> ("edge detected"=w417:bool)  [unwired: 14 in]
    n365 = Compound Arithmetic op=OR(w420, w390, w417) -> (w426:bool)
    n366 = call-poly <instrlib>:"Count Up.vi"("increment"=w399, "reset"=w426) -> ("count out"=w416:u32)  [unwired: 13 in]
    n367 = Equal To 0?(x=w416) -> (x = 0?=w443:bool)
    n368 = Equal?(x=w419, y=w416) -> (x = y?=w442:bool)
    n369 = feedback-in #95(w442) -> ()
    n370 = Decrement(x=w416) -> (x-1=w387:u32)
    n371 = Compound Arithmetic op=OR(w390, w443) -> (w415:bool)
    n372 = xnode ("Memory Read")("Address"=w387) -> ("Data"=w386:bool)  [unwired: 1 in, 1 out]
    n373 = call "SOQPSK Precoder.vi"("Bit In"=w386, "enable"=w397, "input valid"=w399, "reset"=w415) -> ("Alpha Out"=w430:fxp<+/-,3,2>, "output valid"=w429:bool)  [unwired: 9 in, 1 out]
    n374 = feedback #97() -> (w435:bool)  [unwired: 1 in]
    n375 = call "SOQPSK Alpha to IQ.vi"("Alpha in"=w430, "SOQPSK Parameters"=w431, "input valid"=w429, "ready for output"=w435, "reset"=w390) -> ("IQ data out"=w436:T11[], "output valid"=w405:bool, "ready for input"=w434:bool, "error"=w424:bool)  [unwired: 5 in, 2 out]
    n376 = feedback-in #96(w434) -> ()
    n377 = Index Array(array=w436) -> (element #1=w414:T11, element #2=w396:T11)  [unwired: 2 in]
    n378 = Unbundle(w414) -> ("I"=w413:fxp<+/-,18,1>, "Q"=w412:fxp<+/-,18,1>)  [unwired: 1 out]
    n379 = Unbundle(w396) -> ("I"=w411:fxp<+/-,18,1>, "Q"=w410:fxp<+/-,18,1>)  [unwired: 1 out]
    n380 = call "Add AWGN.vi"("real"=w413, "img"=w412, "input valid"=w405, "reset"=w390, "seed"=w394, "scaling factor"=w406, "Output Type Selection"=w403) -> ("output with noise"=w409:u32)  [unwired: 7 in, 1 out]
    n381 = call "Add AWGN.vi"("real"=w411, "img"=w410, "input valid"=w405, "reset"=w390, "seed"=w393, "scaling factor"=w406, "Output Type Selection"=w403) -> ("output with noise"=w408:u32, "output valid"=w385:bool)  [unwired: 7 in]
    n382 = Build Array(w409, w408) -> (w383:u32[])
    n383 = Compound Arithmetic op=AND(invert w435, w385) -> (w440:bool)
    n384 = call <instrlib>:"Synchronous Latch.vi"("clear"=w441, "set"=w440) -> ("out"=w438:bool)  [unwired: 9 in]
    n385 = call <instrlib>:"Synchronous Latch.vi"("clear"=w441, "set"=w424) -> ("out"=w423:bool)  [unwired: 9 in]
    n386 = feedback #98() -> (w382:bool)  [unwired: 1 in]
    n387 = feedback-in #98(w385) -> ()
    n388 = feedback #99() -> (→"write data stream overflow.1":bool)  [unwired: 1 in]
    n389 = feedback-in #99(w438) -> ()
    n390 = feedback #100() -> (→"modulator error.1":bool)  [unwired: 1 in]
    n391 = feedback-in #100(w423) -> ()
    n392 = feedback #101() -> (w402:bool)  [unwired: 1 in]
    n393 = feedback-in #101(w386) -> ()
    n394 = feedback #102() -> (w401:bool)  [unwired: 1 in]
    n395 = feedback-in #102(w399) -> ()
    n396 = feedback #103() -> (w400:u32)  [unwired: 1 in]
    n397 = feedback-in #103(w387) -> ()
    n398 = feedback #104() -> (w398:bool)  [unwired: 1 in]
    n399 = feedback-in #104(w399) -> ()
    n400 = feedback #105() -> (w425:u32[])  [unwired: 1 in]
    n401 = feedback-in #105(w383) -> ()
    n402 = xnode ("FIFO Method Node")("Element"=w402, "Input Valid"=w401) -> ()  [unwired: 1 in, 2 out]
    n403 = xnode ("FIFO Method Node")("Element"=w400, "Input Valid"=w398) -> ()  [unwired: 1 in, 2 out]
    n404 = xnode ("FIFO Method Node")("Element"=w425, "Input Valid"=w382) -> ()  [unwired: 1 in, 2 out]
    n405 = call <vilib>:"U32 Array to Abstract Data Array.vi"("data in"=w383) -> ("data out"=w444:cluster{"Boolean array":bool[]}[])  [unwired: 10 in]
    n406 = call-dynamic "Write.vi"("buffer u32 common"=w446, "reset"=w445, "input valid"=w382, "data in"=w444) -> ("ready for input"=w384:bool)  [unwired: 7 in]
    n407 = feedback-in #97(w384) -> ()
  }
  n408 = timed-loop {
    timing: w29 -> [_]
    timing-out: [_] -> w28
    tunnel: w23 -> [w545]
    stop <- _ stop-if-true
    w528 = T14 2 items=["Idle", "Initial Threshold Detection", "Demodulating"] ("Demodulation Control")
    w530 = T14 0 items=["Idle", "Initial Threshold Detection", "Demodulating"] ("Demodulation Control")
    # "always ready"
    # "1 SPC Buffer read"
    # "Receive IP\n1 SPC @ 160 MHZ = 160M samples/second max"
    n409 = local read "reset rx.1"() -> (w542:bool)
    n410 = local read "reset overflow status.1"() -> (w500:bool)
    n411 = feedback #106() -> (w541:bool)  [unwired: 1 in]
    n412 = feedback-in #106(w542) -> ()
    n413 = feedback #107() -> (w524:bool)  [unwired: 1 in]
    n414 = feedback-in #107("enable aurora debug.1") -> ()
    n415 = feedback #108() -> (w507:u32)  [unwired: 1 in]
    n416 = feedback-in #108("payload length.1") -> ()
    n417 = feedback #109() -> (w533:T3)  [unwired: 1 in]
    n418 = feedback-in #109("symmetric filter coefficients .1") -> ()
    n419 = feedback #110() -> (w535:bool)  [unwired: 1 in]
    n420 = feedback-in #110("enable match filter.1") -> ()
    n421 = feedback #111() -> (w527:i16)  [unwired: 1 in]
    n422 = feedback-in #111("demodulation control.1") -> ()
    n423 = feedback #112() -> (w508:i32)  [unwired: 1 in]
    n424 = feedback-in #112("preamble.1") -> ()
    n425 = feedback #113() -> (w453:bool)  [unwired: 1 in]
    n426 = feedback-in #113(w500) -> ()
    n427 = call-dynamic "Read.vi"("buffer u32 common"=w545, "ready for output"=TRUE, "reset"=w541) -> ("output valid"=w452:bool, "data out"=w543:cluster{"data":bool[]}[])  [unwired: 7 in]
    n428 = Not Equal?(x=w530, y=w527) -> (x != y?=w529:bool)
    n429 = Equal?(x=w527, y=w528) -> (x = y?=w526:bool)
    n430 = call <vilib>:"Abstract Data Array to U32 Array.vi"("data in"=w543) -> ("data out"=w450:u32[])  [unwired: 10 in]
    n431 = Index Array(array=w450) -> (element=w451:u32)  [unwired: 1 in]
    n432 = Split Number(x=w451) -> (hi(x)=w537:u16, lo(x)=w538:u16)
    n433 = Compound Arithmetic op=AND(w452, w529) -> (w495:bool)
    n434 = Compound Arithmetic op=AND(w452, w526) -> (w493:bool)
    n435 = Number To Boolean Array(number=w538) -> (Boolean array=w539:bool[])
    n436 = Number To Boolean Array(number=w537) -> (Boolean array=w540:bool[])
    n437 = Boolean Array To Number(Boolean array=w539) -> (number=w499:fxp<+/-,16,1>)
    n438 = Boolean Array To Number(Boolean array=w540) -> (number=w497:fxp<+/-,16,1>)
    n439 = feedback #114() -> (w498:fxp<+/-,16,1>)  [unwired: 1 in]
    n440 = feedback-in #114(w499) -> ()
    n441 = feedback #115() -> (w496:fxp<+/-,16,1>)  [unwired: 1 in]
    n442 = feedback-in #115(w497) -> ()
    n443 = feedback #116() -> (w494:bool)  [unwired: 1 in]
    n444 = feedback-in #116(w495) -> ()
    n445 = feedback #117() -> (w468:bool)  [unwired: 1 in]
    n446 = feedback-in #117(w493) -> ()
    n447 = call "IQ FIR Filter (33tap).vi"("I data in"=w498, "symmetric filter coefficients"=w533, "Q data in"=w496, "enable"=w535, "input valid"=w494) -> ("I filtered output"=w466:fxp<+/-,16,2>, "Q filtered output"=w464:fxp<+/-,16,2>, "output valid"=w467:bool)  [unwired: 8 in]
    n448 = feedback #118() -> (w465:fxp<+/-,16,2>)  [unwired: 1 in]
    n449 = feedback-in #118(w466) -> ()
    n450 = feedback #119() -> (w461:fxp<+/-,16,2>)  [unwired: 1 in]
    n451 = feedback-in #119(w464) -> ()
    n452 = feedback #120() -> (w462:bool)  [unwired: 1 in]
    n453 = feedback-in #120(w467) -> ()
    n454 = feedback #121() -> (w463:bool)  [unwired: 1 in]
    n455 = feedback-in #121(w468) -> ()
    n456 = call "SOQPSK Preamble Detection.vi"("x real in"=w465, "x im in"=w461, "input valid"=w462, "enable"=w463, "Preamble"=w508) -> ("current threshold"=w502:fxp<+/-,15,15>, "r after preamble"=w470:fxp<+/-,16,1>, "img after preamble"=w472:fxp<+/-,16,1>, "phase valid"=w474:bool, "frequency offset estimation"=w476:fxp<+/-,25,-7>, "phase estimation"=w478:fxp<+/-,24,2>, "estimation valid"=w480:bool)  [unwired: 3 in, 1 out]
    n457 = feedback #122() -> (w469:fxp<+/-,16,1>)  [unwired: 1 in]
    n458 = feedback-in #122(w470) -> ()
    n459 = feedback #123() -> (w471:fxp<+/-,16,1>)  [unwired: 1 in]
    n460 = feedback-in #123(w472) -> ()
    n461 = feedback #124() -> (w473:bool)  [unwired: 1 in]
    n462 = feedback-in #124(w474) -> ()
    n463 = feedback #125() -> (w475:fxp<+/-,25,-7>)  [unwired: 1 in]
    n464 = feedback-in #125(w476) -> ()
    n465 = feedback #126() -> (w477:fxp<+/-,24,2>)  [unwired: 1 in]
    n466 = feedback-in #126(w478) -> ()
    n467 = feedback #127() -> (w479:bool)  [unwired: 1 in]
    n468 = feedback-in #127(w480) -> ()
    n469 = call "SOQPSK Correction.vi"("real input"=w469, "frame length"=w507, "img input"=w471, "input valid"=w473, "frequency offset estimation"=w475, "phase estimation"=w477, "estimation valid"=w479) -> ("real output"=w486:fxp<+/-,33,4>, "img output"=w484:fxp<+/-,33,4>, "output valid"=w483:bool, "reset for IDF"=w488:bool)  [unwired: 5 in]
    n470 = feedback #128() -> (w485:fxp<+/-,33,4>)  [unwired: 1 in]
    n471 = feedback-in #128(w486) -> ()
    n472 = feedback #129() -> (w482:fxp<+/-,33,4>)  [unwired: 1 in]
    n473 = feedback-in #129(w484) -> ()
    n474 = feedback #130() -> (w481:bool)  [unwired: 1 in]
    n475 = feedback-in #130(w483) -> ()
    n476 = feedback #131() -> (w487:bool)  [unwired: 1 in]
    n477 = feedback-in #131(w488) -> ()
    n478 = call "IQ Integrate and Dump Filter (8 samples).vi"("reset"=w487, "input valid"=w481, "img"=w482, "real"=w485) -> ("output valid"=w489:bool, "output"=w492:fxp<+/-,36,7>, "output bit"=w490:bool)  [unwired: 5 in]
    n479 = feedback #132() -> (w491:fxp<+/-,36,7>)  [unwired: 1 in]
    n480 = feedback-in #132(w492) -> ()
    n481 = feedback #133() -> (w460:bool)  [unwired: 1 in]
    n482 = feedback-in #133(w490) -> ()
    n483 = feedback #134() -> (w454:bool)  [unwired: 1 in]
    n484 = feedback-in #134(w489) -> ()
    n485 = case shown="True" w524 {
      tunnel: w451 -> [_ w547]
      tunnel: w452 -> [_ w549]
      tunnel: [_ w550] -> w515
      tunnel: [_ w548] -> w514
      frame False {
      }
      frame True {
        n486 = feedback #135() -> (w546:u32)  [unwired: 1 in]
        n487 = feedback-in #135(w547) -> ()
        n488 = feedback #136() -> (w548:bool)  [unwired: 1 in]
        n489 = feedback-in #136(w549) -> ()
        n490 = xnode ("FIFO Method Node")("Element"=w546, "Input Valid"=w548) -> ("Ready for Input"=w550:bool)  [unwired: 1 in, 1 out]
      }
    }
    n491 = To Fixed-Point(number=w491) -> (fixed-point=w506:fxp<+/-,32,7>)  [unwired: 1 in]
    n492 = Fixed-Point to Integer Cast(1:w506) -> (0:w505:i32)
    n493 = xnode ("FIFO Method Node")("Element"=w505, "Input Valid"=w454) -> ("Ready for Input"=w504:bool)  [unwired: 1 in, 1 out]
    n494 = xnode ("FIFO Method Node")("Element"=w460, "Input Valid"=w454) -> ("Ready for Input"=w503:bool)  [unwired: 1 in, 1 out]
    n495 = xnode ("FIFO Write Using Handshaking")("Element"=w460, "Input Valid"=w454) -> ("Ready for Input"=w455:bool)  [unwired: 1 in, 1 out]
    n496 = feedback #137() -> (w522:bool)  [unwired: 1 in]
    n497 = feedback-in #137(w503) -> ()
    n498 = feedback #138() -> (w518:bool)  [unwired: 1 in]
    n499 = feedback-in #138(w515) -> ()
    n500 = feedback #139() -> (w509:bool)  [unwired: 1 in]
    n501 = feedback-in #139(w504) -> ()
    n502 = feedback #140() -> (w456:bool)  [unwired: 1 in]
    n503 = feedback-in #140(w455) -> ()
    n504 = Compound Arithmetic op=AND(invert w518, w514) -> (w517:bool)
    n505 = Compound Arithmetic op=AND(invert w509, w454) -> (w510:bool)
    n506 = Compound Arithmetic op=AND(invert w522, w454) -> (w521:bool)
    n507 = Compound Arithmetic op=AND(invert w456, w454) -> (w457:bool)
    n508 = call <instrlib>:"Synchronous Latch.vi"("clear"=w453, "set"=w517) -> ("out"=w516:bool)  [unwired: 9 in]
    n509 = call <instrlib>:"Synchronous Latch.vi"("clear"=w453, "set"=w510) -> ("out"=w511:bool)  [unwired: 9 in]
    n510 = call <instrlib>:"Synchronous Latch.vi"("clear"=w453, "set"=w521) -> ("out"=w520:bool)  [unwired: 9 in]
    n511 = call <instrlib>:"Synchronous Latch.vi"("clear"=w453, "set"=w457) -> ("out"=w458:bool)  [unwired: 9 in]
    n512 = feedback #141() -> (→"current threshold.1":fxp<+/-,15,15>)  [unwired: 1 in]
    n513 = feedback-in #141(w502) -> ()
    n514 = feedback #142() -> (→"aurora debug overflow.1":bool)  [unwired: 1 in]
    n515 = feedback-in #142(w516) -> ()
    n516 = feedback #143() -> (→"recovered IQ overflow.1":bool)  [unwired: 1 in]
    n517 = feedback-in #143(w511) -> ()
    n518 = feedback #144() -> (→"demodulated bits overflow.1":bool)  [unwired: 1 in]
    n519 = feedback-in #144(w520) -> ()
    n520 = feedback #145() -> (→"demodulated bits to BER overflow.1":bool)  [unwired: 1 in]
    n521 = feedback-in #145(w458) -> ()
  }
  n522 = timed-loop {
    timing: w19 -> [_]
    timing-out: [_] -> w18
    stop <- _ stop-if-true
    # "bit generation loop"
    n523 = feedback #146() -> (w554:bool)  [unwired: 1 in]
    n524 = feedback-in #146("update bit generation.1") -> ()
    n525 = call <instrlib>:"Detect Rising Edge.vi"("signal"=w554) -> ("edge detected"=w553:bool)  [unwired: 14 in]
    n526 = case shown="True" w554 {
      selector: w554 -> [_ w560]
      tunnel: w553 -> [_ w563]
      frame False {
        # "Don't update"
      }
      frame True {
        # "update"
        n527 = xnode ("FIFO Method Node")("Ready for Output"=TRUE) -> ("Element"=w562:bool, "Output Valid"=w558:bool)  [unwired: 1 in, 1 out]
        n528 = Compound Arithmetic op=AND(w558, w560) -> (w559:bool)
        n529 = call-poly <instrlib>:"Count Up.vi"("increment"=w559, "reset"=w563) -> ("count out"=w556:u32)  [unwired: 13 in]
        "bit stream length.1" <- w556
        n530 = Decrement(x=w556) -> (x-1=w557:u32)
        n531 = case shown="True" w558 {
          tunnel: w557 -> [_ w565]
          tunnel: w562 -> [_ w564]
          frame False {
            # "nothing to write"
          }
          frame True {
            # "write to bit stream memory"
            n532 = xnode ("Memory Write")("Address"=w565, "Data"=w564) -> ()  [unwired: 1 in, 1 out]
          }
        }
      }
    }
  }
  n533 = timed-loop {
    timing: w51 -> [_]
    timing-out: [_] -> w50
    tunnel: w48 -> [w571]
    stop <- _ stop-if-true
    # "bit error rate"
    n534 = xnode ("FIFO Read Using Handshaking")("Ready for Output"=TRUE) -> ("Element"=w570:bool, "Output Valid"=w569:bool)  [unwired: 1 in, 1 out]
    n535 = call "BER 1BPC.vi"("input valid"=w569, "input bits"=w570, "BER"=w571) -> ()  [unwired: 9 in]
  }
  n536 = timed-loop {
    timing: w70 -> [_]
    timing-out: [_] -> w69
    tunnel: w68 -> [w574]
    stop <- _ stop-if-true
    # "Instruction Framework Host Interface"
    n537 = call <instrlib>:"Host Interface.vi"("fifo register bus"=w574, "fifo reg bus ctrl 0"="fifo reg bus ctrl 0") -> ("fifo reg bus status 0"=→"fifo reg bus status 0":u32, "fifo reg bus data 0"=→"fifo reg bus data 0":u64)  [unwired: 12 in]
  }
  n538 = node-c288(w69) -> ()
  n539 = node-c288(w50) -> ()
  n540 = node-c288(w44) -> ()
  n541 = node-c288(w26) -> ()
  n542 = node-c288(w18) -> ()
  n543 = node-c288(w42) -> ()
  n544 = node-c288(w28) -> ()
